vi "Run Pre Build Checks.vi"(0 "NI Build Specification in":refnum<class "NI Build Specification_LV.lvclass">, 11 "error in (no error)":errorcluster) -> (4 "NI Build Specification out":refnum<class "NI Build Specification_LV.lvclass">, 15 "error out":errorcluster)   [LabVIEW 2017, in "CL_G3_VIComponentBuilder.lvlib" / "NI Build Specification_LV.lvclass"]
doc: "Runs the checks necessary to ensure the project passes tests before attempting a build."
uses:
  NI Build Specification_LV.lvclass
  C:/builds/Component BuilderBT/SrcDist/Exports/Exports/Export.lvclass
  Exports/Export.lvclass/Export.ctl
  NI Build Specification_LV.lvclass/NI Build Specification_LV.ctl
  Exports/Accessors/Read Export Build Specification.vi
  Accessors/Read Target Name Containing Build Specs to Build.vi
  Accessors/Read LabVIEW Project SubBuild Spec Order.vi
  Accessors/Read Export's Build Spec Name.vi
  Exports/Accessors/Read Export Config File.vi
  Accessors/Read Build Spec Type.vi
  Exports/Accessors/Read Product Name.vi
  <vilib>/xml/Close Reference(Node).vi
  <resource>/objmgr/DOMUserDefRef.rc
  <vilib>/xml/NI_XML.lvlib
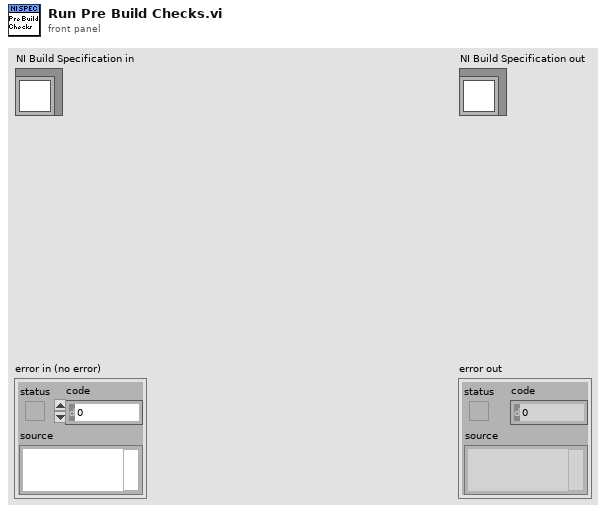
[diagram p1: front panel]
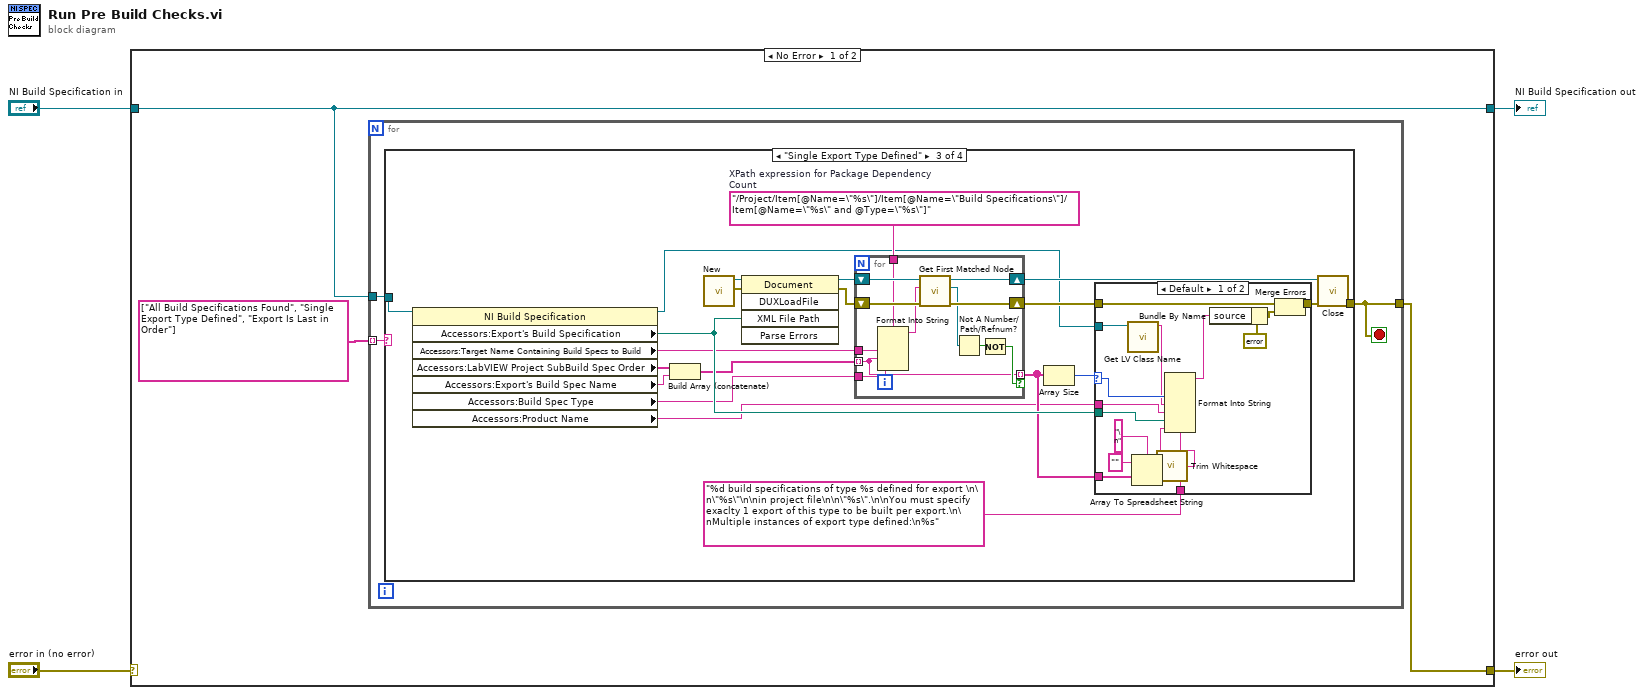
[diagram p0: block diagram]
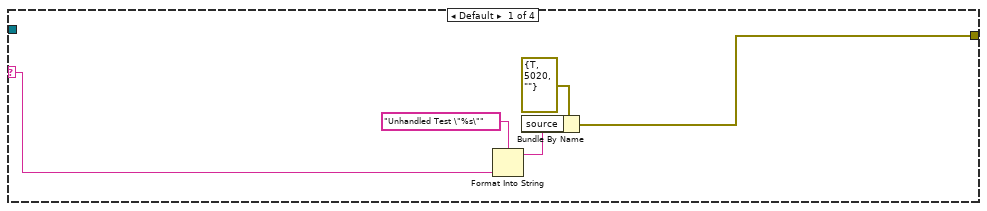
[diagram p2: hidden frame]
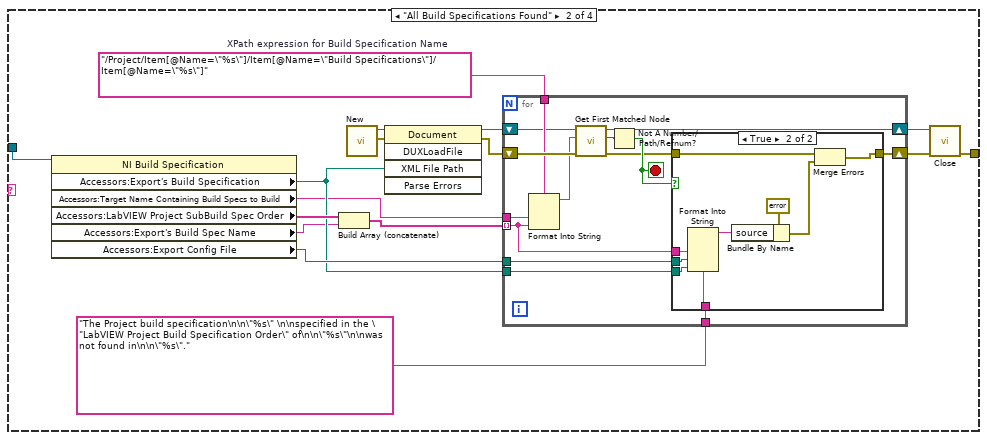
[diagram p3: hidden frame]
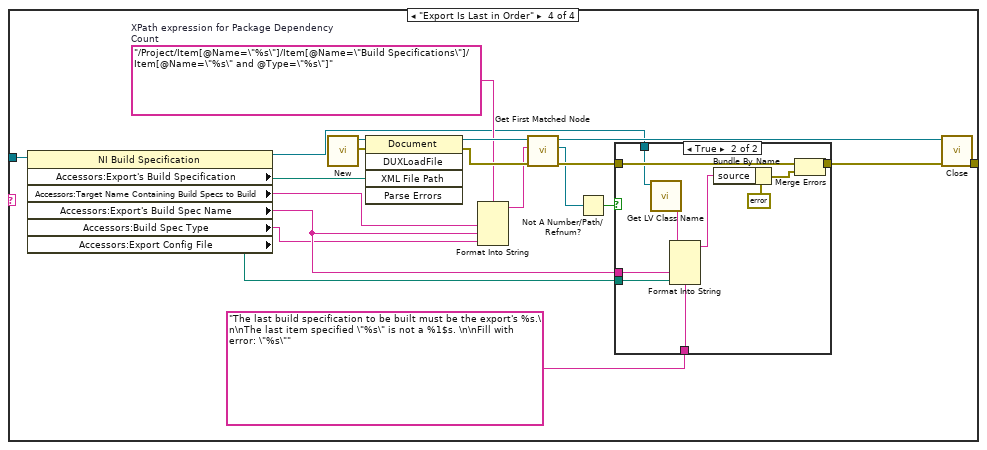
[diagram p6: hidden frame]
diagram:
  n1 = case shown="No Error" "error in (no error)" {
    selector: "error in (no error)" -> [_ w138]
    tunnel: [w5 w138] -> w3
    tunnel: [w6 w137] -> w1
    tunnel: "NI Build Specification in" -> [w6 w137]
    frame No Error {
      n2 = for {
        tunnel: [w9] -> w5
        tunnel: string[] ["All Build Specifications Found", "Single Export Type Defined", "Export Is Last in Order"] -> [w10] mode=indexing
        tunnel: w6 -> [w8]
        stop <- w9 stop-if-true
        n3 = case shown="\"Single Export Type Defined\"" w10 {
          selector: w10 -> [w12 _ _ _]
          tunnel: [w14 w24 w70 w120] -> w9
          tunnel: w8 -> [_ w19 w61 w109]
          frame Default {
            n4 = Format Into String(format string="Unhandled Test \"%s\"", w12) -> (resulting string=w11:string)  [unwired: 2 in, 1 out]
            n5 = Bundle By Name(cluster=errorcluster {"status"=TRUE, "code"=5020, "source"=""} ("error out"), "source"=w11) -> (w14:errorcluster)
          }
          frame "All Build Specifications Found" {
            w30 = "/Project/Item[@Name=\"%s\"]/Item[@Name=\"Build Specifications\"]/Item[@Name=\"%s\"]"  # XPath expression for Build Specification Name
            n6 = property class="NI Build Specification"(reference=w19) -> ("Accessors:Export's Build Specification"=w21:path, "Accessors:Target Name Containing Build Specs to Build"=w18:string, "Accessors:LabVIEW Project SubBuild Spec Order"=w25:string[], "Accessors:Export's Build Spec Name"=w16:string, "Accessors:Export Config File"=w22:path)  [unwired: 1 in, 2 out]
            n7 = Build Array (concatenate)(w25, w16) -> (w17:string[])
            n8 = call <vilib>:"New.vi"() -> ("error out"=w27:errorcluster, "DOM document out"=w26:refnum<k20>)  [unwired: 8 in]
            n9 = invoke class="Document" method="DUXLoadFile"(reference=w26, error in=w27, "XML File Path"=w21) -> (reference out=w28:refnum<k20>, error out=w31:errorcluster)  [unwired: 2 in, 3 out]
            n10 = for {
              tunnel: w30 -> [w44]
              shift-right: [w36] -> w20
              shift-left: w31 -> [w45]
              shift-right: [w42] -> w29
              shift-left: w28 -> [w43]
              tunnel: w17 -> [w33] mode=indexing
              tunnel: "The Project build specification\n\n\"%s\" \n\nspecified in the \"LabVIEW Project Build Specification Order\" of\n\n\"%s\"\n\nwas not found in\n\n\"%s\"." ("format string") -> [w39]
              tunnel: w22 -> [w35]
              tunnel: w21 -> [w34]
              tunnel: w18 -> [w32]
              stop <- w40 stop-if-true
              n11 = Format Into String(format string=w44, w32, w33) -> (resulting string=w37:string)  [unwired: 2 in, 1 out]
              n12 = call <vilib>:"Get First Matched Node.vi"("error in (no error)"=w45, "XPath expression"=w37, "node in"=w43) -> ("error out"=w38:errorcluster, "node result"=w41:refnum<k20>, "node out"=w42:refnum<k20>)  [unwired: 6 in]
              n13 = Not A Number/Path/Refnum?(number/path/refnum=w41) -> (NaN/Path/Refnum?=w40:bool)
              n14 = case shown="True" w40 {
                tunnel: w39 -> [_ w55]
                tunnel: w38 -> [w46 w51]
                tunnel: w33 -> [_ w54]
                tunnel: [w46 w50] -> w36
                tunnel: w35 -> [_ w48]
                tunnel: w34 -> [_ w47]
                frame False {
                }
                frame True {
                  n15 = Format Into String(format string=w55, w54, w48, w47) -> (resulting string=w52:string)  [unwired: 2 in, 1 out]
                  n16 = Bundle By Name(cluster=errorcluster {"status"=TRUE, "code"=0, "source"=""} ("error out"), "source"=w52) -> (w49:errorcluster)
                  n17 = Merge Errors(w51, w49) -> (w50:errorcluster)
                }
              }
            }
            n18 = call-poly <vilib>:"Close.vi"("error in (no error)"=w20, "node"=w29) -> ("error out"=w24:errorcluster)  [unwired: 7 in]
          }
          frame "Single Export Type Defined" {
            w64 = "/Project/Item[@Name=\"%s\"]/Item[@Name=\"Build Specifications\"]/Item[@Name=\"%s\" and @Type=\"%s\"]"  # XPath expression for Package Dependency Count
            n19 = property class="NI Build Specification"(reference=w61) -> (reference out=w60:refnum<class "NI Build Specification_LV.lvclass">, "Accessors:Export's Build Specification"=w65:path, "Accessors:Target Name Containing Build Specs to Build"=w59:string, "Accessors:LabVIEW Project SubBuild Spec Order"=w71:string[], "Accessors:Export's Build Spec Name"=w56:string, "Accessors:Build Spec Type"=w62:string, "Accessors:Product Name"=w58:string)  [unwired: 1 in, 1 out]
            n20 = Build Array (concatenate)(w71, w56) -> (w57:string[])
            n21 = call <vilib>:"New.vi"() -> ("error out"=w73:errorcluster, "DOM document out"=w72:refnum<k20>)  [unwired: 8 in]
            n22 = invoke class="Document" method="DUXLoadFile"(reference=w72, error in=w73, "XML File Path"=w65) -> (reference out=w74:refnum<k20>, error out=w76:errorcluster)  [unwired: 2 in, 3 out]
            n23 = for {
              tunnel: w64 -> [w98]
              shift-right: [w100] -> w68
              shift-left: w76 -> [w105]
              shift-right: [w103] -> w75
              shift-left: w74 -> [w104]
              tunnel: w57 -> [w95] mode=indexing
              tunnel: [w95] -> w63 mode=indexing if=w101
              tunnel: w62 -> [w96]
              tunnel: w59 -> [w94]
              n24 = Format Into String(format string=w98, w94, w95, w96) -> (resulting string=w97:string)  [unwired: 2 in, 1 out]
              n25 = call <vilib>:"Get First Matched Node.vi"("error in (no error)"=w105, "XPath expression"=w97, "node in"=w104) -> ("error out"=w100:errorcluster, "node result"=w99:refnum<k20>, "node out"=w103:refnum<k20>)  [unwired: 6 in]
              n26 = Not A Number/Path/Refnum?(number/path/refnum=w99) -> (NaN/Path/Refnum?=w102:bool)
              n27 = Not(x=w102) -> (.not. x?=w101:bool)
            }
            n28 = Array Size(array=w63) -> (size(s)=w69:i32)
            n29 = case shown="Default" w69 {
              selector: w69 -> [w86 _]
              tunnel: w68 -> [w92 w93]
              tunnel: [w88 w93] -> w67
              tunnel: "%d build specifications of type %s defined for export \n\n\"%s\"\n\nin project file\n\n\"%s\".\n\nYou must specify exaclty 1 export of this type to be built per export.\n\nMultiple instances of export type defined:\n%s" ("format string") -> [w87 _]
              tunnel: w58 -> [w79 _]
              tunnel: w65 -> [w85 _]
              tunnel: w63 -> [w80 _]
              tunnel: w60 -> [w78 _]
              frame Default {
                n30 = call <vilib>:"Get LV Class Name.vi"("object"=w78) -> ("class name"=w77:string)  [unwired: 9 in, 1 out]
                n31 = Array To Spreadsheet String(delimiter (Tab)="\n", array=w80, 3:"" ("format string")) -> (spreadsheet string=w84:string)
                n32 = call <vilib>:"Trim Whitespace.vi"("string"=w84) -> ("trimmed string"=w82:string)  [unwired: 1 in]
                n33 = Format Into String(format string=w87, w86, w77, w79, w85, w82) -> (resulting string=w90:string)  [unwired: 2 in, 1 out]
                n34 = Bundle By Name(cluster=errorcluster {"status"=TRUE, "code"=0, "source"=""} ("error out"), "source"=w90) -> (w89:errorcluster)
                n35 = Merge Errors(w92, w89) -> (w88:errorcluster)
              }
              frame 1 {
              }
            }
            n36 = call-poly <vilib>:"Close.vi"("error in (no error)"=w67, "node"=w75) -> ("error out"=w70:errorcluster)  [unwired: 7 in]
          }
          frame "Export Is Last in Order" {
            w115 = "/Project/Item[@Name=\"%s\"]/Item[@Name=\"Build Specifications\"]/Item[@Name=\"%s\" and @Type=\"%s\"]"  # XPath expression for Package Dependency Count
            n37 = property class="NI Build Specification"(reference=w109) -> (reference out=w108:refnum<class "NI Build Specification_LV.lvclass">, "Accessors:Export's Build Specification"=w116:path, "Accessors:Target Name Containing Build Specs to Build"=w107:string, "Accessors:Export's Build Spec Name"=w112:string, "Accessors:Build Spec Type"=w110:string, "Accessors:Export Config File"=w106:path)  [unwired: 1 in, 1 out]
            n38 = call <vilib>:"New.vi"() -> ("error out"=w122:errorcluster, "DOM document out"=w121:refnum<k20>)  [unwired: 8 in]
            n39 = invoke class="Document" method="DUXLoadFile"(reference=w121, error in=w122, "XML File Path"=w116) -> (reference out=w123:refnum<k20>, error out=w125:errorcluster)  [unwired: 2 in, 3 out]
            n40 = Format Into String(format string=w115, w107, w112, w110) -> (resulting string=w113:string)  [unwired: 2 in, 1 out]
            n41 = call <vilib>:"Get First Matched Node.vi"("error in (no error)"=w125, "XPath expression"=w113, "node in"=w123) -> ("error out"=w119:errorcluster, "node result"=w114:refnum<k20>, "node out"=w124:refnum<k20>)  [unwired: 6 in]
            n42 = Not A Number/Path/Refnum?(number/path/refnum=w114) -> (NaN/Path/Refnum?=w111:bool)
            n43 = case shown="True" w111 {
              tunnel: w119 -> [w126 w136]
              tunnel: [w126 w132] -> w118
              tunnel: "The last build specification to be built must be the export's %s.\n\nThe last item specified \"%s\" is not a %1$s. \n\nFill with error: \"%s\"" ("format string") -> [_ w130]
              tunnel: w112 -> [_ w129]
              tunnel: w106 -> [_ w131]
              tunnel: w108 -> [_ w128]
              frame False {
              }
              frame True {
                n44 = call <vilib>:"Get LV Class Name.vi"("object"=w128) -> ("class name"=w127:string)  [unwired: 9 in, 1 out]
                n45 = Format Into String(format string=w130, w127, w129, w131) -> (resulting string=w134:string)  [unwired: 2 in, 1 out]
                n46 = Bundle By Name(cluster=errorcluster {"status"=TRUE, "code"=0, "source"=""} ("error out"), "source"=w134) -> (w133:errorcluster)
                n47 = Merge Errors(w136, w133) -> (w132:errorcluster)
              }
            }
            n48 = call-poly <vilib>:"Close.vi"("error in (no error)"=w118, "node"=w124) -> ("error out"=w120:errorcluster)  [unwired: 7 in]
          }
        }
      }
    }
    frame Error {
    }
  }
  "error out" <- w3
  "NI Build Specification out" <- w1
